vi "FT10_Log TDMS Values.vi"(8 "error in":errorcluster, 9 "Waveform filename":string, 10 "Log Cluster in":T4, 11 "Log Loop Cluster in":T1) -> (0 "error out":errorcluster, 3 "Log Loop Cluster out":T1)   [LabVIEW 2015]
uses:
  Controls/Control_Log Cluster.ctl
  Controls/Control_Log Time.ctl
  Controls/Control_Log Waveform Cluster.ctl
  Controls/Control_Log Analysis Cluster.ctl
  Controls/Control_Log Loop Cluster.ctl
  Controls/Control_Log TDMS Filename.ctl
  Controls/Control_Log t0.ctl
  <vilib>/Waveform/WDTOps.llb/WDT Number of Waveform Samples DBL.vi
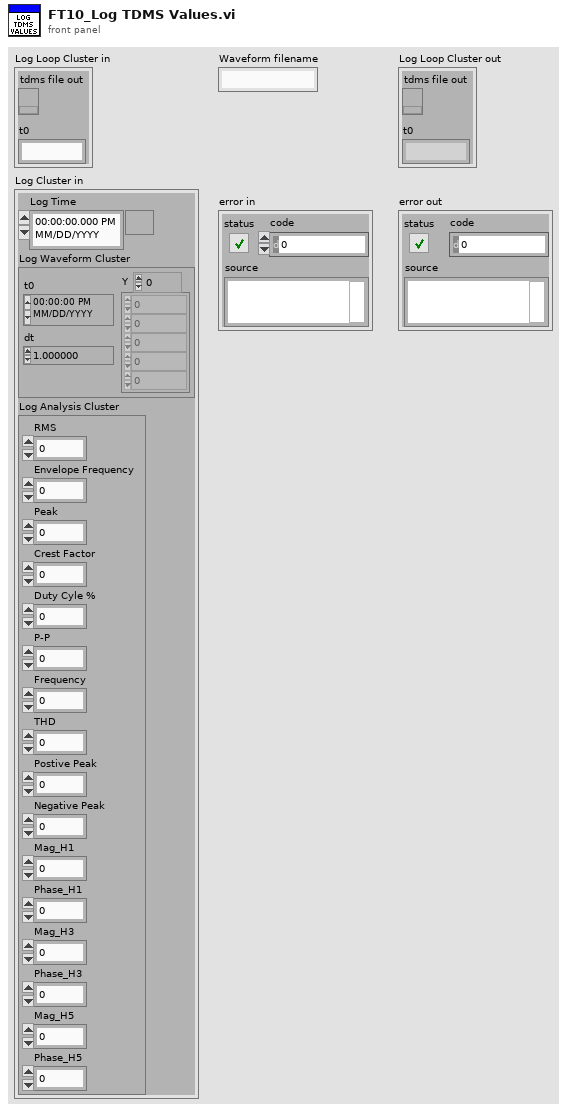
[diagram p1: front panel]
types:
  T1 = typedef "Control_Log Loop Cluster.ctl" = cluster{"tdms file out":T2, "t0":T3}
  T2 = typedef "Control_Log TDMS Filename.ctl" = refnum<k34>
  T3 = typedef "Control_Log t0.ctl" = string
  T4 = typedef "Control_Log Cluster.ctl" = cluster{"Log Time":T5, "Log Waveform Cluster":T6, "Log Analysis Cluster":T7}
  T5 = typedef "Control_Log Time.ctl" = timestamp
  T6 = typedef "Control_Log Waveform Cluster.ctl" = waveform(dbl)
  T7 = typedef "Control_Log Analysis Cluster.ctl" = cluster{"RMS":dbl, "Envelope Frequency":dbl, "Peak":dbl, "Crest Factor":dbl, "Duty Cyle %":dbl, "P-P":dbl, "Frequency":dbl, "THD":dbl, "Postive Peak":dbl, "Negative Peak":dbl, "Mag_H1":dbl, "Phase_H1":dbl, "Mag_H3":dbl, "Phase_H3":dbl, "Mag_H5":dbl, "Phase_H5":dbl}
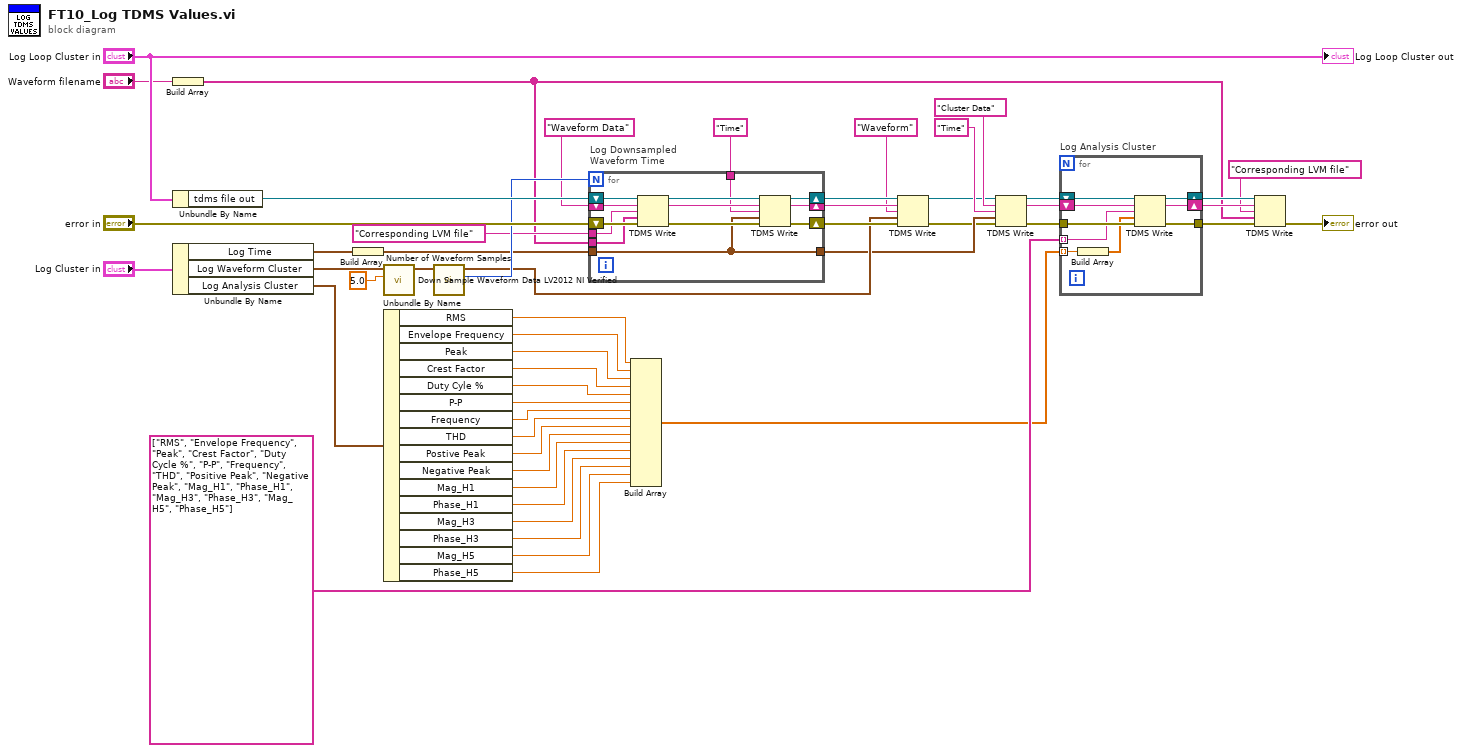
[diagram p0: block diagram]
diagram:
  n1 = Build Array("Waveform filename") -> (w2:string[])
  n2 = Unbundle By Name("Log Loop Cluster in") -> ("tdms file out"=w46:T2)
  n3 = Unbundle By Name("Log Cluster in") -> ("Log Time"=w42:T5, "Log Waveform Cluster"=w49:T6, "Log Analysis Cluster"=w16:T7)
  n4 = Build Array(w42) -> (w41:T5[])
  n5 = call "Down Sample Waveform Data LV2012 NI Verified.vi"("Desired Sampling Rate"=5.0, "Waveform in"=w49) -> ("Waveform out"=w48:waveform(dbl))  [unwired: 8 in, 1 out]
  n6 = Unbundle By Name(w16) -> ("RMS"=w32:dbl, "Envelope Frequency"=w31:dbl, "Peak"=w30:dbl, "Crest Factor"=w29:dbl, "Duty Cyle %"=w28:dbl, "P-P"=w27:dbl, "Frequency"=w26:dbl, "THD"=w25:dbl, "Postive Peak"=w24:dbl, "Negative Peak"=w23:dbl, "Mag_H1"=w22:dbl, "Phase_H1"=w21:dbl, "Mag_H3"=w20:dbl, "Phase_H3"=w19:dbl, "Mag_H5"=w18:dbl, "Phase_H5"=w17:dbl)
  n7 = call-poly <vilib>:"Number of Waveform Samples.vi"("waveform in"=w48) -> ("number of samples"=w45:i32, "waveform out"=w36:waveform(dbl))  [unwired: 8 in, 1 out]
  n8 = for "Log Downsampled Waveform Time" {
    N: w45 -> [_]
    tunnel: "Corresponding LVM file" ("channel name(s) in (Untitled)") -> [w62]
    tunnel: w41 -> [w54]
    shift-right: [w59] -> w39
    shift-left: "Waveform Data" ("group name in (Untitled)") -> [w65]
    shift-right: [w60] -> w40
    shift-left: w46 -> [w64]
    shift-right: [w56] -> w38
    shift-left: "error in" -> [w63]
    tunnel: [w54] -> w33
    tunnel: "Time" ("channel name(s) in (Untitled)") -> [w55]
    tunnel: w2 -> [w53]
    n9 = TDMS Write(0:w64, 5:w65, 7:w62, 9:w53, 11:w63) -> (4:w61:refnum<k34>, 6:w58:string, 15:w57:errorcluster)  [unwired: 1 in, 1 out]
    n10 = TDMS Write(0:w61, 5:w58, 7:w55, 9:w54, 11:w57) -> (4:w60:refnum<k34>, 6:w59:string, 15:w56:errorcluster)  [unwired: 1 in, 1 out]
  }
  n11 = Build Array(w32, w31, w30, w29, w28, w27, w26, w25, w24, w23, w22, w21, w20, w19, w18, w17) -> (w12:dbl[])
  n12 = TDMS Write(0:w40, 5:w39, 7:"Waveform" ("channel name(s) in (Untitled)"), 9:w36, 11:w38) -> (4:w10:refnum<k34>, 15:w9:errorcluster)  [unwired: 1 in, 2 out]
  n13 = TDMS Write(0:w10, 5:"Cluster Data" ("group name in (Untitled)"), 7:"Time" ("channel name(s) in (Untitled)"), 9:w33, 11:w9) -> (4:w15:refnum<k34>, 6:w14:string, 15:w11:errorcluster)  [unwired: 1 in, 1 out]
  n14 = for "Log Analysis Cluster" {
    shift-right: [w73] -> w4
    shift-left: w15 -> [w74]
    shift-right: [w71] -> w3
    shift-left: w14 -> [w72]
    tunnel: w11 -> [w70]
    tunnel: [w69] -> w6
    tunnel: w12 -> [w68] mode=indexing
    tunnel: string[] ["RMS", "Envelope Frequency", "Peak", "Crest Factor", "Duty Cycle %", "P-P", "Frequency", "THD", "Positive Peak", "Negative Peak", "Mag_H1", "Phase_H1", "Mag_H3", "Phase_H3", "Mag_H5", "Phase_H5"] ("channel name(s) in (Untitled)") -> [w66] mode=indexing
    n15 = Build Array(w68) -> (w67:dbl[])
    n16 = TDMS Write(0:w74, 5:w72, 7:w66, 9:w67, 11:w70) -> (4:w73:refnum<k34>, 6:w71:string, 15:w69:errorcluster)  [unwired: 1 in, 1 out]
  }
  n17 = TDMS Write(0:w4, 5:w3, 7:"Corresponding LVM file" ("channel name(s) in (Untitled)"), 9:w2, 11:w6) -> (15:→"error out":errorcluster)  [unwired: 1 in, 3 out]
  "Log Loop Cluster out" <- "Log Loop Cluster in"
